vi "ErrorHandler.vi"(8 "error in (no error)":errorcluster, 11 "queue out":refnum<queue>) -> (0 "error out":errorcluster)   [LabVIEW 2019, in "Prueba10.lvclass"]
uses:
  Prueba10.lvclass
  Controles/MessageP10.ctl
  Controles/EstadosP10.ctl
  <vilib>/ErrorRing/Error Ring.xnode
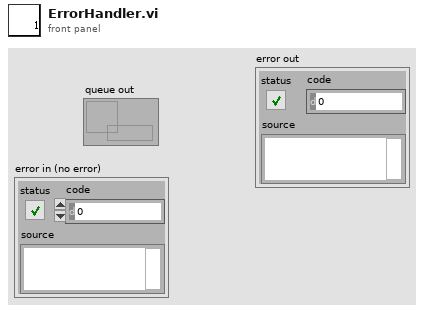
[diagram p1: front panel]
types:
  T1 = typedef "Prueba10.lvclass/EstadosP10.ctl" = enum16{"DetieneInstrumentos", "InicializarInstrumentos", "LeerArchivoConfiguracion", "Error", "inicio", "configurarTabla", "FrecAmp1", "FrecAmp2", "FrecAmp3", "suma_resta", "calcularVref", "iniciarGEN", "iniciarGEN_2", "reset-NivRefEnsayo", "guardaVref", "monitoreo", "monitoreo_2", "ingresaMediciones", "guardarMediciones", "detenerGEN", "cumplimiento", "listo_evaluar", "evaluar", "final", "salir"}
  T2 = typedef "Prueba10.lvclass/MessageP10.ctl" = cluster{"Estados":T1, "Data":variant}
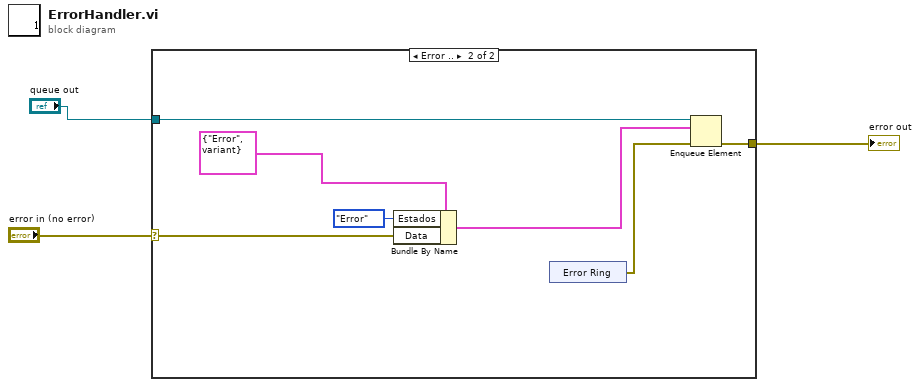
[diagram p0: block diagram]
diagram:
  n1 = case shown="Error .." "error in (no error)" {
    selector: "error in (no error)" -> [w4 w9]
    tunnel: "queue out" -> [_ w10]
    tunnel: [w4 w11] -> w2
    frame No Error {
    }
    frame Error {
      n2 = Bundle By Name(cluster=T2 {"Estados"=enum."Error", "Data"=variant} ("element"), "Estados"=EstadosP10."Error", "Data"=w9) -> (w8:T2)
      n3 = xnode "Error Ring"() -> ("error out"=w7:errorcluster)
      n4 = Enqueue Element(queue=w10, element=w8, error in (no error)=w7) -> (error out=w11:errorcluster)  [unwired: 1 in, 2 out]
    }
  }
  "error out" <- w2
